vi "Configure Device.vi"(8 "error in":errorcluster, 11 "Configurable Device in":refnum<class "Configurable Device.lvclass">) -> (0 "error out":errorcluster, 2 "CfgDataOut":string, 3 "Configurable Device out":refnum<class "Configurable Device.lvclass">, 4 "SP":dbl, 5 "Settable?":bool)   [LabVIEW 2014, in "Device.lvlib" / "Configurable Device.lvclass"]
uses:
  Configurable Device.lvclass
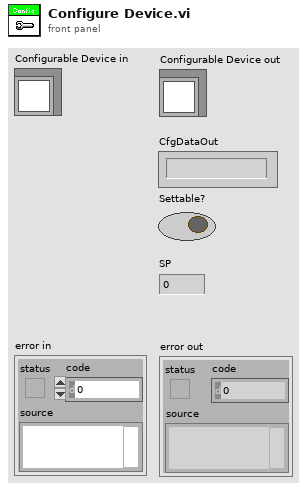
[diagram p1: front panel]
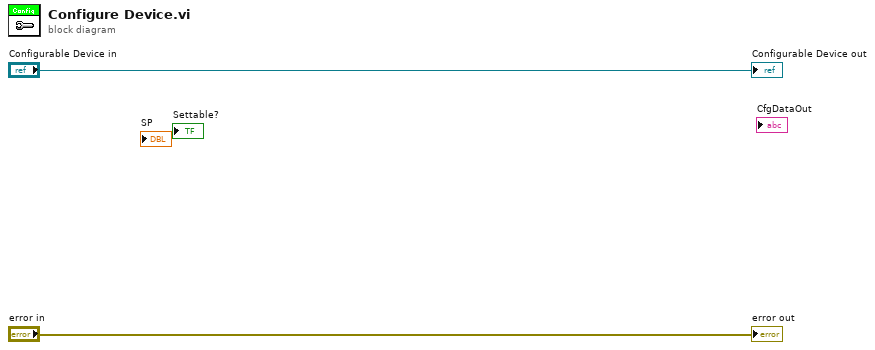
[diagram p0: block diagram]
diagram:
  "error out" <- "error in"
  "Configurable Device out" <- "Configurable Device in"
